vi "get_by_asset.path.vi"() -> (2 "path":string)   [LabVIEW 2020, in "Run.lvclass"]
uses:
  Run.lvclass
  Run.lvclass/Run.ctl
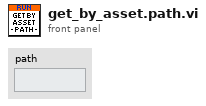
[diagram p1: front panel]
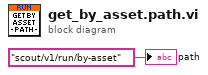
[diagram p0: block diagram]
diagram:
  "path" <- "scout/v1/run/by-asset"
